vi "Uninstall Components.vi"(8 "error in (no error)":errorcluster, 11 "Configuration in":T1) -> (0 "error out":errorcluster, 2 "Deleted Components":path[](array[path]), 3 "Configuration out":T1)   [LabVIEW 2011, in "LVH-Build-Tools.lvlib"]
uses:
  LVH-Build-Tools.lvlib
  Type Defs/Configuration.ctl
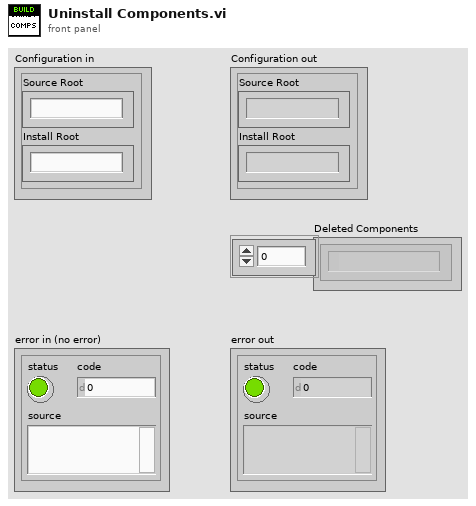
[diagram p1: front panel]
types:
  T1 = typedef "LVH-Build-Tools.lvlib/Configuration.ctl" = cluster{"Source Root":string, "Install Root":string, "Components":string[], "Ignore":string[]}
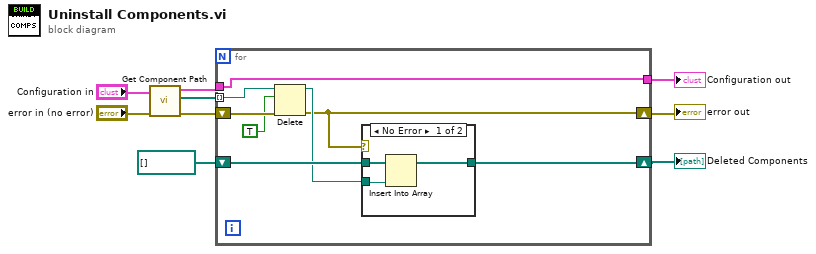
[diagram p0: block diagram]
diagram:
  n1 = call "Get Component Path.vi"("Error In"="error in (no error)", "Configuration"="Configuration in") -> ("Error Out"=w5:errorcluster, "Component Install Paths"=w4:path[], "Configuration"=w7:T1)  [unwired: 7 in]
  n2 = for {
    tunnel: w7 -> [w14]
    shift-right: [w12] -> w1
    shift-left: path[] [] -> [w17]
    shift-right: [w11] -> w2
    shift-left: w5 -> [w16]
    tunnel: w4 -> [w10] mode=indexing
    tunnel: [w14] -> w3
    n3 = Delete(path (use dialog)=w10, entire hierarchy (F)=TRUE, error in=w16) -> (deleted path=w13:path, error out=w11:errorcluster)  [unwired: 2 in, 1 out]
    n4 = case shown="No Error" w11 {
      tunnel: w17 -> [w20 w21]
      tunnel: w13 -> [w19 _]
      tunnel: [w18 w21] -> w12
      frame No Error {
        n5 = Insert Into Array(array=w20, new element=w19) -> (w18:path[])  [unwired: 1 in]
      }
      frame Error {
      }
    }
  }
  "error out" <- w2
  "Configuration out" <- w3
  "Deleted Components" <- w1
